vi "Read.vi"(8 "error in (no error)":errorcluster, 11 "Double Float.lvclass_340760 in":refnum<class "Abs_Complex Single Float.lvclass">) -> (0 "error out":errorcluster, 2 "Value":T1, 3 "Double Float.lvclass_340760 out":refnum<class "Abs_Complex Single Float.lvclass">)   [LabVIEW 2021, in "Abs_Complex Single Float.lvclass"]
uses:
  Abs_Complex Single Float.lvclass
  Support/Type.ctl
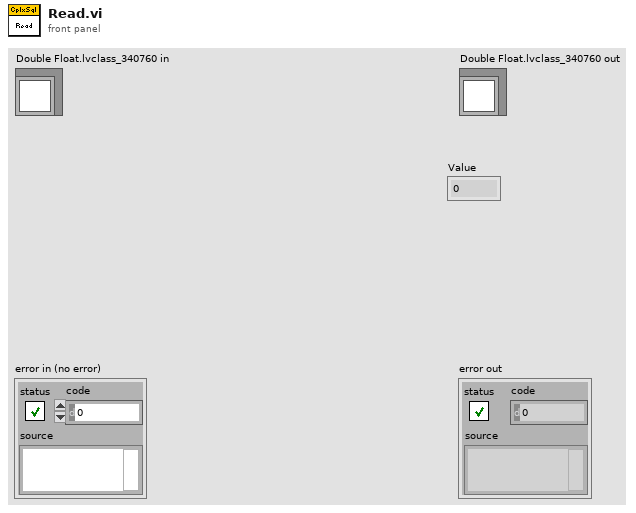
[diagram p1: front panel]
types:
  T1 = typedef "Abs_Complex Single Float.lvclass/Type.ctl" = csg
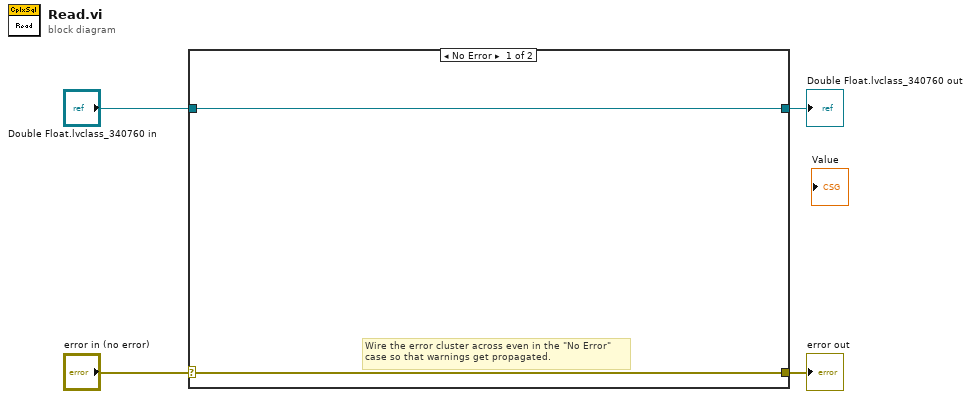
[diagram p0: block diagram]
diagram:
  n1 = case shown="No Error" "error in (no error)" {
    selector: "error in (no error)" -> [w5 w8]
    tunnel: [w5 w8] -> w3
    tunnel: [w6 w7] -> w1
    tunnel: "Double Float.lvclass_340760 in" -> [w6 w7]
    frame No Error {
      # "Wire the error cluster across even in the \"No Error\"\ncase so that warnings get propagated."
    }
    frame Error {
    }
  }
  "error out" <- w3
  "Double Float.lvclass_340760 out" <- w1
